vi "Read Parameter VS Channels.vi"(8 "error in (no error)":errorcluster, 10 "To HWOut Buf in":dbl[](array[numeric]), 11 "Label Settings":T1 {"Words"."Param Setting"."Num Bits" min=1 max=32; "Words"."Param Setting"."Start Bit" min=8 max=31; "Words"."Block Data Refs"."Data Reference" format="%.0x"; "Label" format="%.0o"}) -> (0 "error out":errorcluster, 2 "To HWOut Buf out":dbl[](array[numeric]), 3 "Label Settings":T1 {"Words"."Param Setting"."Num Bits" min=1 max=32; "Words"."Param Setting"."Start Bit" min=8 max=31; "Words"."Block Data Refs"."Data Reference" format="%.0x"; "Label" format="%.0o"})   [LabVIEW 2016, in "Ballard Arinc-429 Engine.lvlib"]
uses:
  Ballard Arinc-429 Engine.lvlib
  RT Controls/RT Label Settings.ctl
  Shared/Controls and Global/Label.ctl
  Shared/Controls and Global/transferPeriod.ctl
  RT Controls/Driver Data.ctl
  RT Controls/RT Word Settings.ctl
  <vilib>/NI Veristand/Custom Device API/Block Data Reference.ctl
  <vilib>/NI Veristand/Custom Device API/Data Reference.ctl
  RT Controls/RT Param Setting.ctl
  Shared/Controls and Global/Start Bit.ctl
  Shared/Controls and Global/Number of Bits.ctl
  Shared/Controls and Global/TransferType.ctl
  <vilib>/NI Veristand/Custom Device API/Global Data Refs.vi
  <vilib>/NI Veristand/Custom Device API/Custom Device API.lvlib
  Shared/Ballard Arinc-429 Shared.lvlib
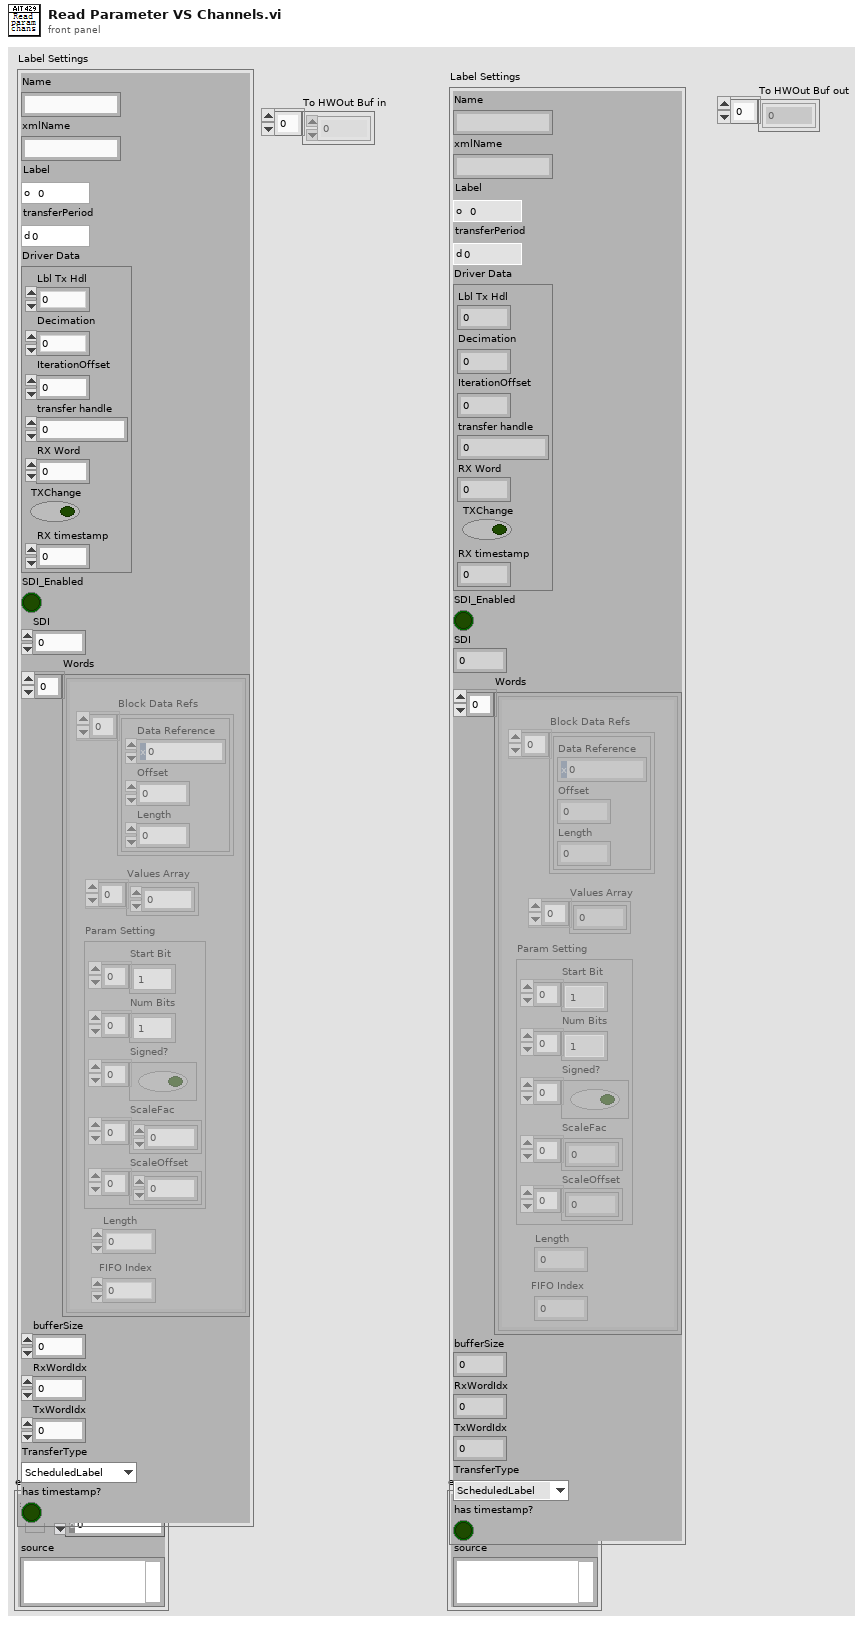
[diagram p1: front panel]
types:
  T1 = typedef "Ballard Arinc-429 Engine.lvlib/RT Label Settings.ctl" = cluster{"Name":string, "xmlName":string, "Label":T2, "transferPeriod":T3, "Driver Data":T4, "SDI_Enabled":bool, "SDI":u8, "Words":T5[], "bufferSize":u32, "RxWordIdx":i32, "TxWordIdx":i32, "TransferType":T11, "has timestamp?":bool}
  T2 = typedef "Ballard Arinc-429 Shared.lvlib/Label.ctl" = u8
  T3 = typedef "Ballard Arinc-429 Shared.lvlib/transferPeriod.ctl" = u32
  T4 = typedef "Ballard Arinc-429 Engine.lvlib/Driver Data.ctl" = cluster{"Lbl Tx Hdl":u32, "Decimation":i32, "IterationOffset":i32, "transfer handle":u32, "RX Word":u32, "TXChange":bool, "RX timestamp":dbl}
  T5 = typedef "Ballard Arinc-429 Engine.lvlib/RT Word Settings.ctl" = cluster{"Block Data Refs":T6[], "Values Array":dbl[], "Length":i32, "FIFO Index":i32, "Param Setting":T8}
  T6 = typedef "Custom Device API.lvlib/Block Data Reference.ctl" = cluster{"Data Reference":T7, "Offset":u64, "Length":u64}
  T7 = typedef "Custom Device API.lvlib/Data Reference.ctl" = i32
  T8 = typedef "Ballard Arinc-429 Engine.lvlib/RT Param Setting.ctl" = cluster{"Start Bit":T9[], "Num Bits":T10[], "Signed?":bool[], "ScaleFac":dbl[], "ScaleOffset":dbl[]}
  T9 = typedef "Ballard Arinc-429 Shared.lvlib/Start Bit.ctl" = i32
  T10 = typedef "Ballard Arinc-429 Shared.lvlib/Number of Bits.ctl" = i32
  T11 = typedef "Ballard Arinc-429 Shared.lvlib/TransferType.ctl" = enum16{"ScheduledLabel", "Acyclic", "Block", "Strobe"}
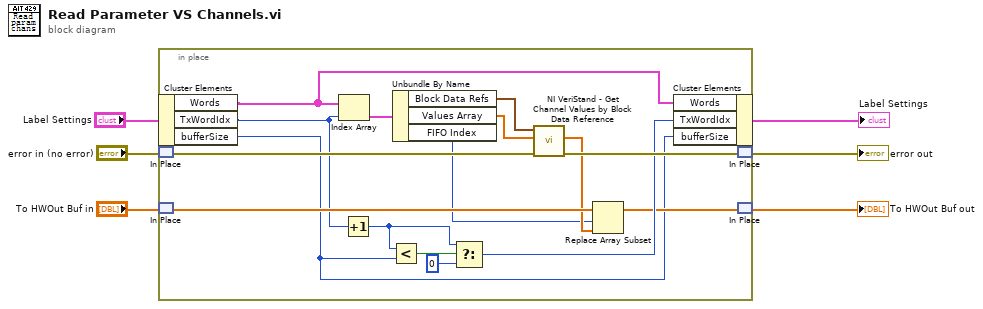
[diagram p0: block diagram]
diagram:
  n1 = in-place {
    n2 = in-place-cluster #1("Label Settings") -> ("Words"=w16:T5[], "TxWordIdx"=w12:i32, "bufferSize"=w9:u32)
    n3 = in-place-match #2("error in (no error)") -> (w17:errorcluster)
    n4 = in-place-match #3("To HWOut Buf in") -> (w13:dbl[])
    n5 = Index Array(array=w16, index=w12) -> (element=w21:T5)
    n6 = Increment(x=w12) -> (x+1=w8:i32)
    n7 = Less?(x=w8, y=w9) -> (x < y?=w20:bool)
    n8 = Unbundle By Name(w21) -> ("Block Data Refs"=w22:T6[], "Values Array"=w11:dbl[], "FIFO Index"=w7:i32)
    n9 = Select(t=w8, s=w20, f=0) -> (s? t:f=w15:i32)
    n10 = call <vilib>:"NI VeriStand - Get Channel Values by Block Data Reference.vi"("error in (no error)"=w17, "Values Array in"=w11, "Block Data Ref"=w22) -> ("error out"=w18:errorcluster, "Values Array out"=w10:dbl[])  [unwired: 6 in, 1 out]
    n11 = Replace Array Subset(array=w13, new element=w10, index=w7) -> (w14:dbl[])
    n12 = in-place-cluster #1("Words"=w16, "TxWordIdx"=w15, "bufferSize"=w9) -> (→"Label Settings":T1)
    n13 = in-place-match #2(w18) -> (→"error out":errorcluster)
    n14 = in-place-match #3(w14) -> (→"To HWOut Buf out":dbl[])
  }
